vi "getActivation.vi"(3 "toCopyTo":sgl[][](array[numeric]), 4 "layer":u32, 5 "ptr":i64, 6 "error in (no error)":errorcluster) -> (0 "toCopyTo 2":sgl[][](array[numeric]), 1 "ptr out":i64, 2 "error out":errorcluster)   [LabVIEW 2016, in "CNet.lvlib"]
uses:
  CNet.lvlib
  Users/jg754/Documents/Visual Studio 2015/Projects/CLearn/x64/Release/CLearn.dll
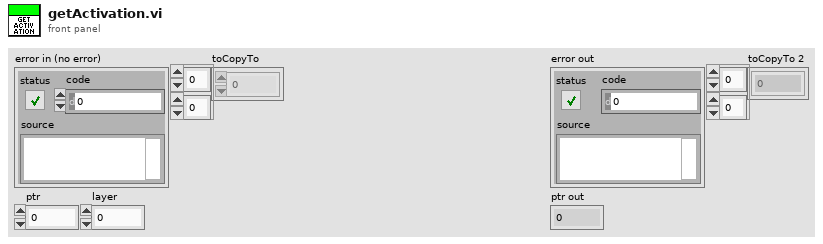
[diagram p1: front panel]
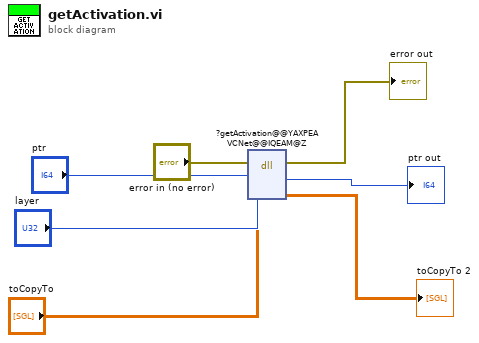
[diagram p0: block diagram]
diagram:
  n1 = dll-call lib="C:/Users/jg754/Documents/Visual Studio 2015/Projects/CLearn/x64/Release/CLearn.dll" fn="?getActivation@@YAXPEAVCNet@@IQEAM@Z"(error in="error in (no error)", "ptr"="ptr", "layer"="layer", "toCopyTo"="toCopyTo") -> (error out=→"error out":errorcluster, "ptr"=→"ptr out":i64, "toCopyTo"=→"toCopyTo 2":sgl[][])  [unwired: 4 in, 1 out]
